vi "libssh2_session_disconnect.vi"(8 "error in (no error)":errorcluster, 10 "description":string, 11 "session":T1) -> (0 "error out":errorcluster, 3 "return value":i32)   [LabVIEW 2013, in "libssh2.lvlib"]
doc: "Sends a disconnect message to the remote host associated with <B>session</B>."
uses:
  libssh2.lvlib
  Session Refnum.ctl
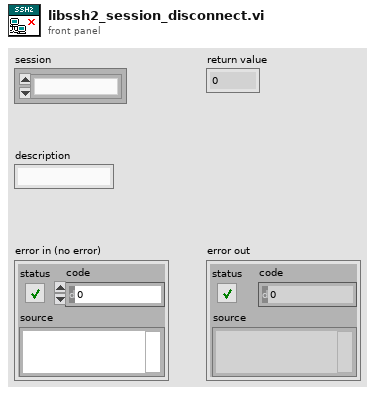
[diagram p1: front panel]
types:
  T1 = typedef "libssh2.lvlib/Session Refnum.ctl" = refnum<k1>
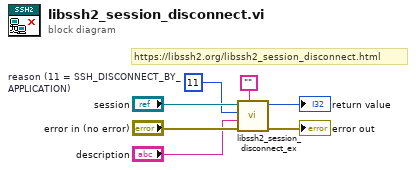
[diagram p0: block diagram]
diagram:
  w4 = 11  # reason (11 = SSH_DISCONNECT_BY_APPLICATION)
  # "https://libssh2.org/libssh2_session_disconnect.html"
  n1 = call "libssh2_session_disconnect_ex.vi"("lang"="", "error in (no error)"="error in (no error)", "description"="description", "reason"=w4, "session"="session") -> ("error out"=→"error out":errorcluster, "return value"=→"return value":i32)  [unwired: 5 in]
